vi "Line Configuration Dialog.vi"(8 "error in":errorcluster, 9 "engine configuration in":refnum<class "engine configuration.lvclass">, 10 "tag bus configurable plugin module configuration":refnum<class "Increment configuration.lvclass">, 11 "Line":T2) -> (0 "error out":errorcluster, 1 "success":bool, 2 "changed":bool, 3 "Mappings out":T1)   [LabVIEW 2015, in "Increment editor node.lvclass"]
doc: "A dialog for allowing a user to specify the values of a new line."
uses:
  Increment editor node.lvclass
  module/configuration/Line.ctl
  <vilib>/NI/Tag Bus Module Framework/channel/TBM channel.lvclass
  Mappings.ctl
  Map.ctl
  <vilib>/NI/Module Execution Interface/Engine Configuration/engine configuration.lvclass
  module/configuration/Increment configuration.lvclass
  <vilib>/NI/DCAF UI Toolkit/Controls/DCAF UI Elements.lvlib
panel:
  out "errors":string
  in  "Increment Name":string
  in  "cancel":bool
  in  "ok":bool
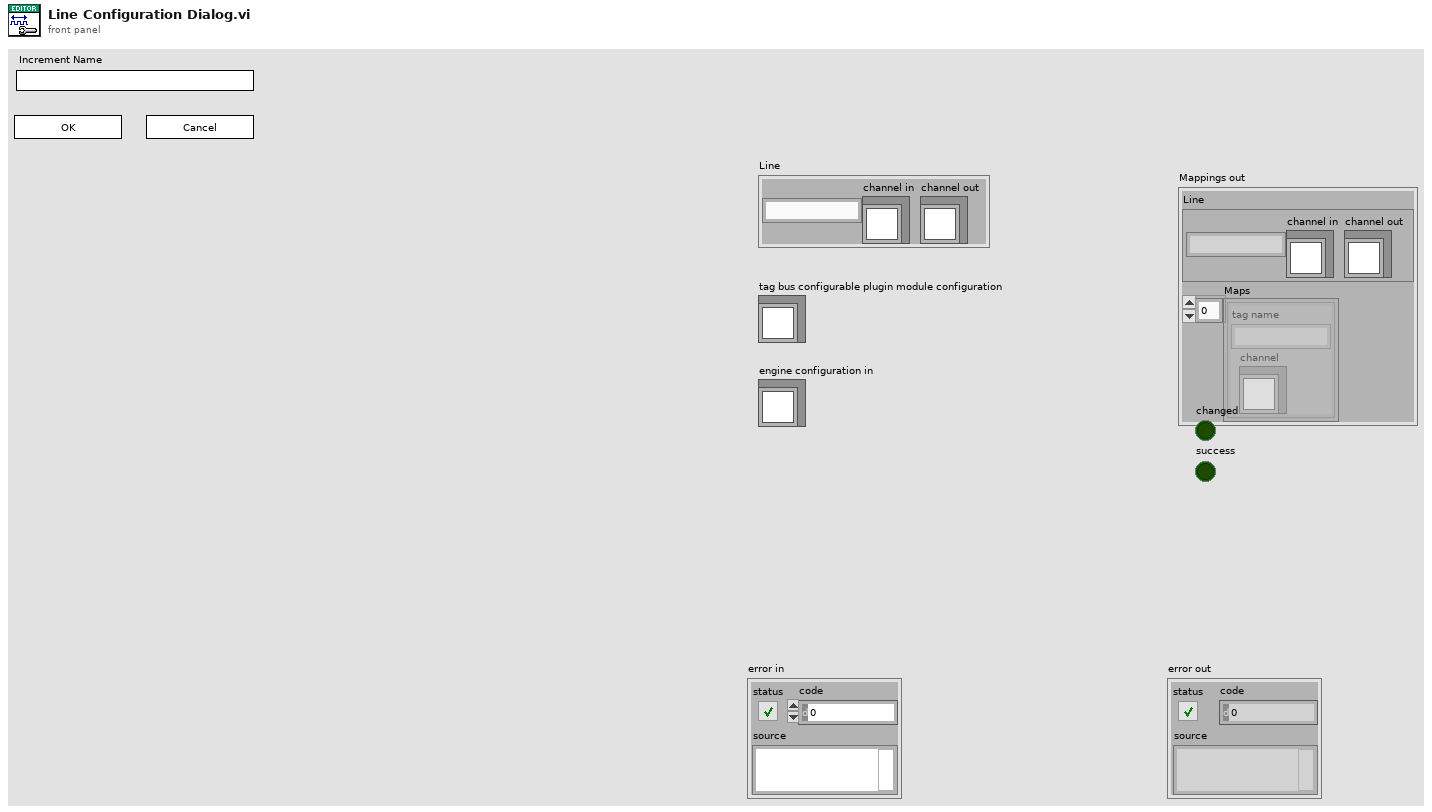
[diagram p1: front panel]
types:
  T1 = typedef "Increment editor node.lvclass/Mappings.ctl" = cluster{"Line":T2, "Maps":T3[]}
  T2 = typedef "Increment configuration.lvclass/Line.ctl" = cluster{"Name":string, "channel in":refnum<class "TBM channel.lvclass">, "channel out":refnum<class "TBM channel.lvclass">}
  T3 = typedef "Increment editor node.lvclass/Map.ctl" = cluster{"channel":refnum<class "TBM channel.lvclass">, "tag name":string}
  T4 = enum8{"Enabled", "Disabled", "Disabled and Grayed Out"}
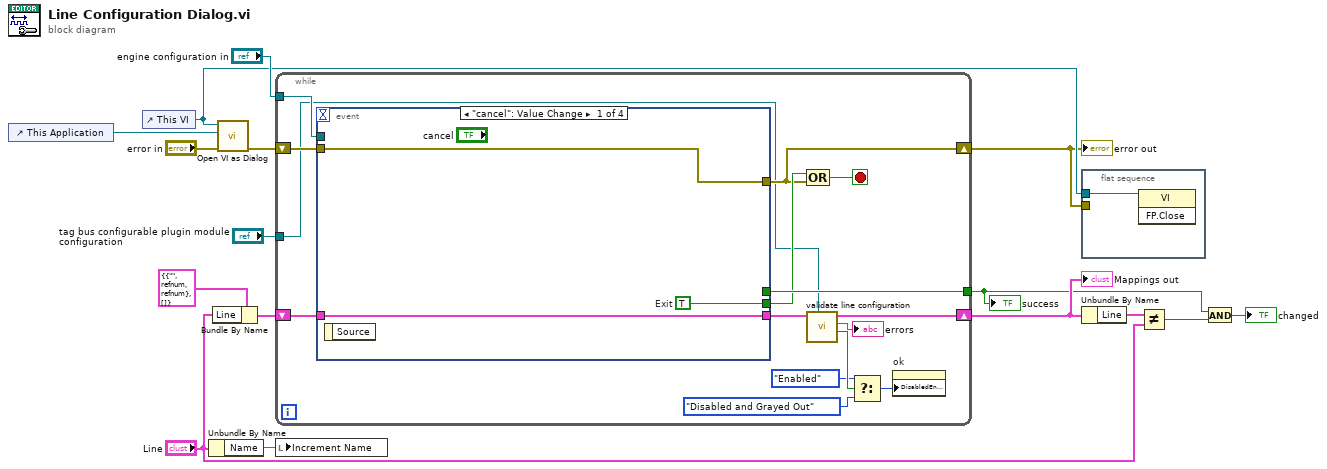
[diagram p0: block diagram]
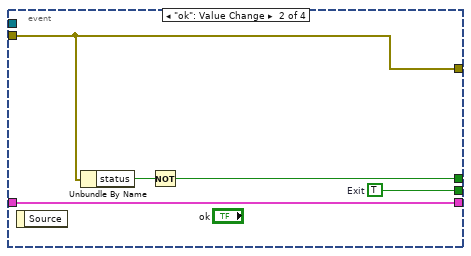
[diagram p2: hidden frame]
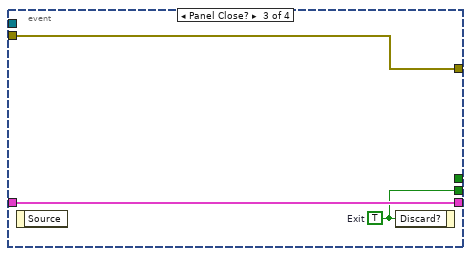
[diagram p3: hidden frame]
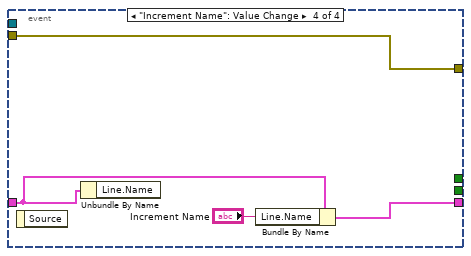
[diagram p4: hidden frame]
diagram:
  n1 = control-ref of="This Application"() -> (w12:refnum<vi>)
  n2 = control-ref of="This VI"() -> (w8:refnum<vi>)
  n3 = Unbundle By Name("Line") -> ("Name"=w3:string)
  n4 = Bundle By Name(cluster=T1 {"Line"={"Name"="", "channel in"=refnum, "channel out"=refnum}, "Maps"=[]} ("Mappings out"), "Line"="Line") -> (w15:T1)
  n5 = call <vilib>:"Open VI as Dialog.vi"("error in (no error)"="error in", "This Application"=w12, "VI in"=w8) -> ("error out"=w10:errorcluster)  [unwired: 8 in]
  n6 = while {
    shift-right: [w23] -> w6
    shift-left: w10 -> [w30]
    tunnel: [w29] -> w5
    shift-right: [w24] -> w13
    shift-left: w15 -> [w26]
    tunnel: "engine configuration in" -> [w31]
    tunnel: "tag bus configurable plugin module configuration" -> [w18]
    stop <- w27 stop-if-true
    n7 = event shown="[0] \"cancel\": Value Change" {
      selector: _ -> [_ _ _ _]
      dyn-events: _ -> [_ _ _ _]
      timeout: _ -> [_ _ _ _]
      tunnel: w31 -> [_ _ _ _]
      tunnel: w30 -> [w34 w37 w42 w46]
      tunnel: [w34 w37 w42 w46] -> w23
      tunnel: [_ w35 _ _] -> w29
      tunnel: [w32 w38 w40 _] -> w28
      tunnel: w26 -> [w33 w39 w41 w44]
      tunnel: [w33 w39 w41 w45] -> w25
      event "cancel": Value Change {
        w32 = TRUE  # Exit
        n8 = event-data() -> ()  [unwired: 1 in, 1 out]
      }
      event "ok": Value Change {
        w38 = TRUE  # Exit
        n9 = event-data() -> ()  [unwired: 1 in, 1 out]
        n10 = Unbundle By Name(w37) -> ("status"=w36:bool)
        n11 = Not(x=w36) -> (.not. x?=w35:bool)
      }
      event Panel Close? {
        w40 = TRUE  # Exit
        n12 = event-data() -> ()  [unwired: 1 in, 1 out]
        n13 = event-data("Discard?"=w40) -> ()  [unwired: 1 in, 1 out]
      }
      event "Increment Name": Value Change {
        n14 = event-data() -> ()  [unwired: 1 in, 1 out]
        n15 = Unbundle By Name(w44) -> ()  [unwired: 1 out]
        n16 = Bundle By Name(cluster=w44, "Line.Name"="Increment Name") -> (w45:T1)
      }
    }
    n17 = Compound Arithmetic op=OR(w28, w23) -> (w27:bool)
    n18 = call "validate line configuration.vi"("Module Config"=w18, "Mappings in"=w25) -> ("valid?"=w22:bool, "errors"=→"errors":string, "Mappings out"=w24:T1)  [unwired: 7 in]
    n19 = Select(t=T4."Enabled" ("Disabled"), s=w22, f=T4."Disabled and Grayed Out") -> (s? t:f=w19:T4)
    n20 = property on="ok" class="Bool"("DisabledEnum"=w19) -> ()  [unwired: 2 in, 2 out]
  }
  "error out" <- w6
  "success" <- w5
  "Mappings out" <- w13
  n21 = local write "Increment Name"(w3) -> ()
  n22 = flat-sequence {
    tunnel: w6 -> [_]
    tunnel: w8 -> [w47]
    frame #0 {
      n23 = invoke class="VI" method="FP.Close"(reference=w47) -> ()  [unwired: 2 in, 3 out]
    }
  }
  n24 = Unbundle By Name(w13) -> ("Line"=w14:T2)
  n25 = Not Equal?(x=w14, y="Line") -> (x != y?=w1:bool)
  n26 = And(x=w5, y=w1) -> (x .and. y?=→"changed":bool)
